vi "Installer Post-Install Action-OLD.vi"() -> (0 "error out":errorcluster)   [LabVIEW 2020]
uses:
  <vilib>/Utility/sysdir.llb/System Directory Type.ctl
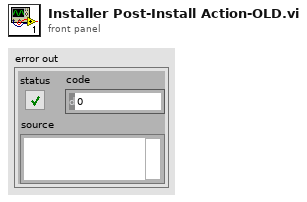
[diagram p1: front panel]
types:
  T1 = typedef "System Directory Type.ctl" = i32
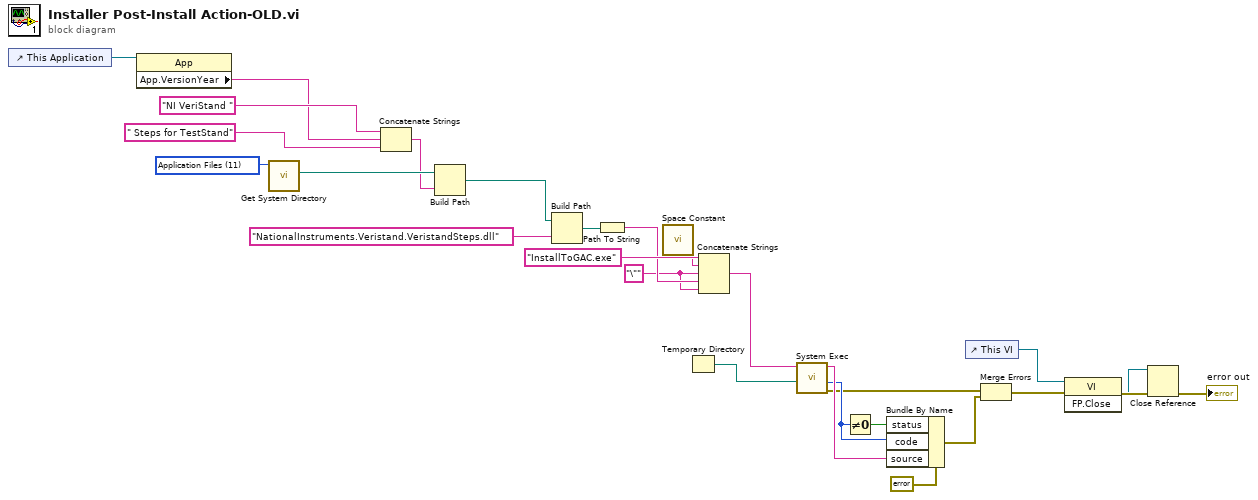
[diagram p0: block diagram]
diagram:
  w14 = T1 11 items=["User Home"=0, "User Desktop"=1, "User Documents"=2, "User Application Data"=3, "User Preferences"=4, "User Temporary"=5, "Public Documents"=6, "Public Application Data"=7, "Public Preferences"=8, "Public Cache"=13, "System Core Libraries"=9, "System Installed Libraries"=10, "Application Files"=11, "Boot Volume Root"=12] ("system directory type")
  w19 = "\"" ("string")
  n1 = control-ref of="This Application"() -> (w3:refnum<vi>)
  n2 = property class="App"(reference=w3) -> ("App.VersionYear"=w2:string)  [unwired: 1 in, 2 out]
  n3 = call <vilib>:"Get System Directory.vi"("system directory type"=w14) -> ("system directory"=w15:path)  [unwired: 10 in]
  n4 = Concatenate Strings("NI VeriStand ", w2, " Steps for TestStand" ("string")) -> (w12:string)
  n5 = Build Path(base path=w15, name or relative path=w12) -> (appended path=w13:path)
  n6 = Build Path(base path=w13, name or relative path="NationalInstruments.Veristand.VeristandSteps.dll" ("command line")) -> (appended path=w24:path)
  n7 = Path To String(path=w24) -> (string=w20:string)
  n8 = call <vilib>:"Space Constant.vi"() -> ("String"=w25:string)
  n9 = Temporary Directory() -> (w17:path)
  n10 = Concatenate Strings("InstallToGAC.exe" ("command line"), w25, w19, w20, w19) -> (w18:string)
  n11 = call <vilib>:"System Exec.vi"("working directory"=w17, "command line"=w18) -> ("error out"=w7:errorcluster, "return code"=w8:i32, "standard output"=w9:string)  [unwired: 6 in, 1 out]
  n12 = Not Equal To 0?(x=w8) -> (x != 0?=w10:bool)
  n13 = Bundle By Name(cluster=errorcluster {"status"=FALSE, "code"=0, "source"=""} ("error constant"), "status"=w10, "code"=w8, "source"=w9) -> (w6:errorcluster)
  n14 = control-ref of="This VI"() -> (w23:refnum<vi>)
  n15 = Merge Errors(w7, w6) -> (w5:errorcluster)
  n16 = invoke class="VI" method="FP.Close"(reference=w23, error in=w5) -> (reference out=w21:refnum<vi>, error out=w22:errorcluster)  [unwired: 1 in, 1 out]
  n17 = Close Reference(reference=w21, error in (no error)=w22) -> (error out=→"error out":errorcluster)
